vi "ExposeOnSetValue.vi"(8 "Requires Response":bool, 9 "Message":T2 {"Message Type" items=["Error"=1, "Warning"=2, "Create"=4, "Destroy"=8, "Invoke"=16, "Get"=32, "Set"=64, "Response"=128]}, 10 "HandlerID":string, 11 "Expose Info":T1) -> (3 "Response":variant)   [LabVIEW 2017]
uses:
  ExposeMessage.ctl
  Events/ExposeMessageType.ctl
  Mapper/ExposeObjectMapNamepathData.ctl
  Mapper/ExposeMapperDataTypeEnum.ctl
  Mapper/ExposeObjectMapContainerTypeEnum.ctl
  ExposeInfo.ctl
  C:/Code/CMCryoSysCode/Expose/COM/CSCom/CSCom/bin/Release/CSCom.dll
  COM/CSCom/CSCom/bin/Release/CSCom.dll
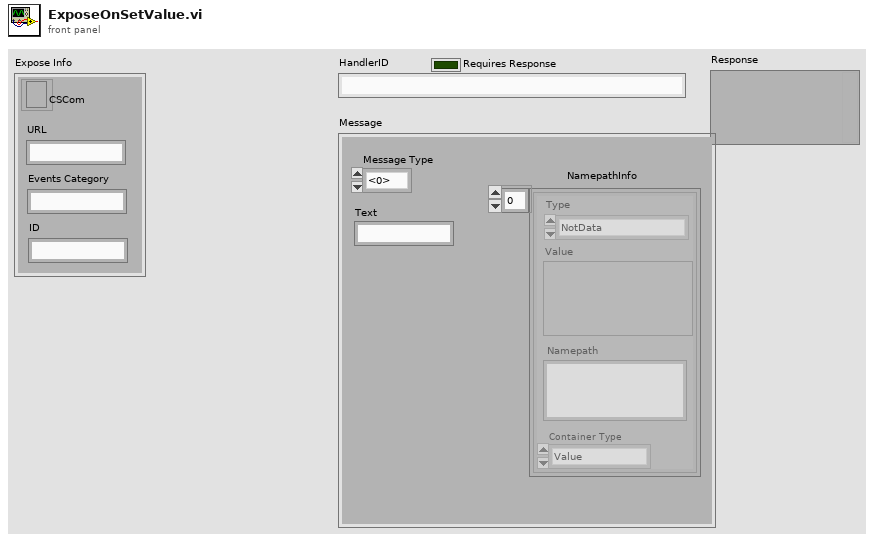
[diagram p1: front panel]
types:
  T1 = typedef "ExposeInfo.ctl" = cluster{"CSCom":refnum<k24>, "URL":string, "Events Category":string, "ID":string}
  T2 = typedef "ExposeMessage.ctl" = cluster{"Message Type":T3, "Text":string, "NamepathInfo":T4[]}
  T3 = typedef "ExposeMessageType.ctl" = i32
  T4 = typedef "ExposeObjectMapNamepathData.ctl" = cluster{"Type":T5, "Value":variant, "Namepath":string, "Container Type":T6}
  T5 = typedef "ExposeMapperDataTypeEnum.ctl" = enum16{"NotData", "int8", "byte", "int16", "uint16", "int32", "uint32", "int64", "uint64", "Single", "Double", "String", "Boolean", "Container"}
  T6 = typedef "ExposeObjectMapContainerTypeEnum.ctl" = enum16{"Value", "Array", "Waveform", "NetContainer"}
  T7 = typedef "ExposeDataType.ctl" = cluster{"Values":variant, "ParameterBindingInfo":variant}
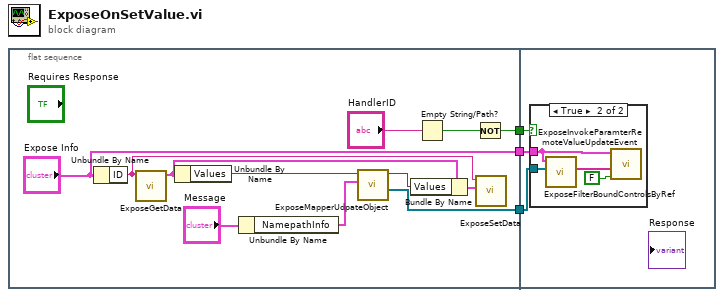
[diagram p0: block diagram]
diagram:
  n1 = flat-sequence {
    tunnel: [w8] -> w3
    tunnel: [w7] -> w2
    tunnel: ["Expose Info"] -> w1
    tunnel: w3 -> [w18]
    tunnel: w2 -> [w17]
    tunnel: w1 -> [w16]
    frame #0 {
      n2 = Unbundle By Name("Expose Info") -> ("ID"=w13:string)
      n3 = call "ExposeGetData.vi"("ExposeID"=w13) -> ("ExposeDataType"=w12:T7)  [unwired: 9 in, 1 out]
      n4 = Unbundle By Name(w12) -> ("Values"=w4:variant)
      n5 = Unbundle By Name("Message") -> ("NamepathInfo"=w14:T4[])
      n6 = call "ExposeMapperUdpateObject.vi"("Object Map"=w14, "Type (or value to update)"=w4) -> ("Updated Controls"=w7:refnum<vi>[], "Value"=w6:variant)  [unwired: 8 in]
      n7 = Bundle By Name(cluster=w12, "Values"=w6) -> (w11:T7)
      n8 = Empty String/Path?(string/path="HandlerID") -> (empty?=w10:bool)
      n9 = Not(x=w10) -> (.not. x?=w8:bool)
      n10 = call "ExposeSetData.vi"("ExposeDataType"=w11, "ExposeID"=w13) -> ()  [unwired: 10 in]
    }
    frame #1 {
      n11 = case shown="True" w18 {
        tunnel: w17 -> [_ w22]
        tunnel: w16 -> [_ w21]
        frame False {
        }
        frame True {
          n12 = call "ExposeFilterBoundControlsByRef.vi"("Controls to Filter"=w22, "Expose Info"=w21) -> ("Bound Control Names"=w20:string[])  [unwired: 8 in, 1 out]
          n13 = call "ExposeInvokeParamterRemoteValueUpdateEvent.vi"("Invoke Value Labview Value Update event"=FALSE, "Names"=w20, "Expose Info"=w21) -> ()  [unwired: 9 in]
        }
      }
    }
  }
